vi "DDS220_xc_umn_new.vi"() -> ()   [LabVIEW 2015]
uses:
  <vilib>/Analysis/baseanly.llb/Mean (DBL).vi
  <vilib>/Instr/_visa.llb/VISA Configure Serial Port (Instr).vi
  Pixis_FSRS_new/Labview VIs/Stanford Research 830/Public/Data/Read (1 Parameter).vi
  <vilib>/Utility/file.llb/Write To Spreadsheet File (DBL).vi
  <vilib>/Analysis/NI_AALBase.lvlib
  Pixis_FSRS_new/Labview VIs/Stanford Research 830/Stanford Research 830.lvlib
panel:
  in  "Vy input":dbl
  in  "Vx input":dbl
  in  "Move 2D Mirror":bool
  in  "MG17Motor":refnum<k7>(container)
  in  "Serial":i32=94868093
  out "Thor error in readout":errorcluster
  in  "Thor error in (no error)":errorcluster
  out "Boolean":bool
  out "Waveform Graph":dbl[](graph)=[-3.576299999999999e-07, 9.735509166666665e-07, -8.543369166666667e-07, -1.3311782499999997e-06, 2.582899166666667e-07, -1.5497290833333338e-06, 3.715376083333334e-06, -9.934158333333333e-07, -6.159184166666667e-07, -7.947341666666668e-07, -5.960483333333331e-07, -6.357897500000001e-07, -8.543380833333334e-07, 3.377623333333333e-07, -4.967065833333332e-07, -7.748691666666666e-07, -1.1126248333333334e-06, 1.3113100833333334e-06, -1.6888085833333337e-06, -8.145998333333333e-07, -1.7086741666666665e-06, 1.45038675e-06, -1.033152583333333e-06, -7.152597500000001e-07, -8.543379999999999e-07, 7.549975833333334e-07, 2.0663075833333334e-06, -1.7682825000000001e-06, -3.1789166666666676e-07, 9.934167499999999e-07, 1.8080217499999998e-06, -1.4305205000000001e-06, -7.3512925e-07, 2.3444625e-06, -5.761805833333333e-07, 2.0861760000000002e-06, 5.761800000000001e-07, 4.0332687499999995e-06, 1.0530233333333335e-06, 1.1523649166666668e-06, 1.1921008333333334e-06, -1.7881241666666663e-07, 2.2252532499999997e-06, 4.768409166666669e-07, 2.185515833333333e-06, 2.3245900833333336e-06, 4.5697000000000005e-07, 1.2119715833333334e-06, -8.146023333333334e-07, 1.7484133333333331e-06, 3.6359025833333332e-06, 2.980246e-06, 1.7285456666666667e-06, 2.8212999999999996e-06, 5.086294e-06, 4.808134083333333e-06, 3.814720916666667e-06, 4.768400833333334e-06, 4.669061000000001e-06, 5.6624715e-06, 7.212209166666667e-06, 1.1364680000000002e-05, 7.967199166666664e-06, 9.199042499999999e-06, 1.0311664166666666e-05, 1.4484019166666666e-05, 1.6093358333333332e-05, 2.0603458333333332e-05, 2.094121666666667e-05, 2.4616841666666666e-05, 2.870973333333333e-05, 2.8828933333333334e-05, 3.323970833333333e-05, 3.6935225e-05, 4.146518333333334e-05, 4.456464166666667e-05, 5.8452574999999995e-05, 6.701593333333332e-05, 8.302974166666666e-05, 9.667923333333334e-05, 0.00010430865, 0.00011529566666666664, 0.00013200541666666667, 0.00014907225000000002, 0.00016401308333333333, 0.00017162258333333334, 0.00018302691666666662, 0.00017992758333333332, 0.00016901983333333332, 0.00015932408333333334, 0.00014724416666666665, 0.00013774725, 0.00012362083333333331, 0.00011342816666666667, 0.00010422908333333334, 8.1599225e-05, 6.351909166666666e-05, 5.539285833333333e-05, 4.4524900000000005e-05, 3.888233333333333e-05, 3.757101666666667e-05, 3.92797e-05, 3.643850833333333e-05, 3.0795925e-05, 2.5669866666666666e-05, 2.0166358333333336e-05, 1.8159649999999995e-05, 1.3272034166666667e-05, 1.3788616666666667e-05, 1.38879575e-05, 1.4742300000000001e-05, 1.0808380833333335e-05, 8.2850935e-06, 9.556669166666668e-06, 7.410888333333332e-06, 6.258529166666666e-06, 4.271688416666667e-06, 5.9406249999999996e-06, 5.920766666666666e-06, 3.2186668333333334e-06, 3.9537975e-06, 6.794973250000001e-06, 6.238653333333333e-06, 5.1657625000000005e-06, 2.3643309166666665e-06, 1.966964e-06, 3.7948526666666665e-06, 5.304841833333333e-06, 4.311425083333332e-06, 3.616038416666667e-06, 2.40406775e-06, 1.6888091666666666e-06, 4.212084333333333e-06, 3.178937666666667e-06, 3.0398556666666672e-06, 1.3709143333333332e-06, 7.152594999999999e-07, 2.284862666666667e-06, 8.146010833333332e-07, 1.9272292499999995e-06, 2.1259103333333337e-06, 3.159062666666667e-06, -5.36446e-07, 1.0132839999999999e-06, 1.0728908333333333e-06, -5.165766666666667e-07, 1.5497284999999996e-06, 1.1722341666666662e-06, 3.794851750000001e-06, 3.973675000000048e-08, 1.0728899999999999e-06, 1.0530215833333335e-06, 1.2715725833333337e-06, 2.4636706666666665e-06, 2.1060426666666664e-06, -2.384209166666666e-07, 1.9868385833333334e-06, 3.3577483333333332e-06, 3.9736666666666353e-08, -6.755207499999998e-07, 2.0066975833333333e-06, 3.9736645e-06, 8.344708333333334e-07, 3.0994578333333333e-06, 1.5298624166666668e-06, 2.4835408333333335e-06, 2.145781e-06, 2.88090675e-06, 2.8809068333333336e-06, 1.1920974999999993e-07, 3.5564320833333337e-06, 2.7815666666666668e-06, 2.1259160000000003e-06, 8.940750000000001e-07, -2.76169575e-06, 3.6756387499999998e-06, 5.761815833333333e-07, -8.146014166666668e-07, 8.940749999999999e-07, -1.788150833333334e-07, -9.338119166666668e-07, 1.0927573333333334e-06, 1.27157425e-06, -1.1722292500000002e-06, 1.2318368333333332e-06, -4.172325e-07, 2.2848560000000004e-06, 1.3709118333333336e-06, 2.7616977500000003e-06, 3.337880083333333e-06, -9.934159166666668e-07, -1.5894266666666665e-07, 3.7749766666666664e-07, -7.152651666666667e-07, 9.139435833333334e-07, -1.986808333333333e-08, -4.3710175000000006e-07, 1.5298618333333338e-06, -1.291440833333333e-06, 1.2715725000000002e-06]
  in  "Shutter Position":bool=TRUE
  out "Status":string="Shutter Open"
  out "Numeric 2":i32=1
  in  "error out 3":errorcluster
  out "error out 2":errorcluster
  out "Current position":dbl=18.1998
  in  "move":bool
  in  "flow control 2":u16(ring) items=["None"=0, "XON/XOFF"=1, "RTS/CTS"=2, "DTR/DSR"=4]
  in  "stop bits 2":u16(ring)=10 items=["1.0"=10, "1.5"=15, "2.0"=20]
  in  "parity 2":u16(ring) items=["None", "Odd", "Even", "Mark", "Space"]
  in  "data bits 2":u16=8 min=5 max=8 step=1
  in  "VISA resource name 3":refnum<visa-resource-name>="GPIB0::8::INSTR"
  in  "baud rate 2":u32=9600
  in  "Start Position":dbl=17.8
  out "read buffer":string="-2.86104e-006\r"
  out "Numeric":dbl=14.0
  out "Array 2":dbl[](array[numeric])=[17.8019, 17.8038, 17.8058, 17.8078, 17.8098, 17.8118, 17.8138, 17.8157, 17.8177, 17.8199, 17.8219, 17.8237, 17.8258, 17.8278, 17.8298, 17.8318, 17.8337, 17.8358, 17.8378, 17.8398, 17.8418, 17.8438, 17.8458, 17.8478, 17.8497, 17.8518, 17.8538, 17.8558, 17.8578, 17.8598, 17.8618, 17.8638, 17.8658, 17.8678, 17.8698, 17.8718, 17.8737, 17.8759, 17.8778, 17.8799, 17.8818, 17.8838, 17.8858, 17.8878, 17.8898, 17.8918, 17.8938, 17.8958, 17.8978, 17.8996, 17.9018, 17.9038, 17.9058, 17.9077, 17.9098, 17.9118, 17.9138, 17.9159, 17.9177, 17.9197, 17.9218, 17.9238, 17.9258, 17.9278, 17.9298, 17.9318, 17.9338, 17.9357, 17.9378, 17.9397, 17.9419, 17.9438, 17.9458, 17.9478, 17.9499, 17.9518, 17.9538, 17.9559, 17.9579, 17.9596, 17.9618, 17.9637, 17.9658, 17.9678, 17.9698, 17.9718, 17.9738, 17.9759, 17.9777, 17.9801, 17.9818, 17.9838, 17.9858, 17.9878, 17.9898, 17.9918, 17.9938, 17.9957, 17.9978, 18.0, 18.0018, 18.0038, 18.0057, 18.0078, 18.0098, 18.0118, 18.0138, 18.0157, 18.0178, 18.0199, 18.0218, 18.0238, 18.0258, 18.0278, 18.0298, 18.0318, 18.0338, 18.0358, 18.0378, 18.0401, 18.0418, 18.0438, 18.0458, 18.0478, 18.0498, 18.0518, 18.0538, 18.0557, 18.0578, 18.06, 18.0618, 18.0638, 18.0658, 18.0677, 18.0698, 18.0718, 18.0738, 18.0758, 18.0778, 18.0796, 18.0818, 18.0838, 18.0857, 18.0878, 18.0898, 18.0918, 18.0937, 18.0958, 18.0978, 18.0998, 18.1018, 18.1038, 18.1058, 18.1078, 18.1098, 18.1118, 18.1138, 18.1159, 18.1178, 18.1198, 18.1218, 18.1237, 18.1257, 18.1277, 18.1297, 18.1318, 18.1338, 18.1356, 18.1378, 18.1398, 18.1418, 18.1437, 18.1457, 18.1478, 18.1498, 18.1518, 18.1538, 18.1558, 18.1577, 18.1598, 18.1618, 18.1637, 18.1658, 18.1678, 18.1698, 18.1718, 18.1738, 18.1758, 18.1778, 18.1798, 18.1818, 18.1838, 18.1858, 18.1878, 18.1898, 18.1917, 18.1937, 18.1958, 18.1977, 18.1998]
  out "Array":dbl[](array[numeric])=[-3.576299999999999e-07, 9.735509166666665e-07, -8.543369166666667e-07, -1.3311782499999997e-06, 2.582899166666667e-07, -1.5497290833333338e-06, 3.715376083333334e-06, -9.934158333333333e-07, -6.159184166666667e-07, -7.947341666666668e-07, -5.960483333333331e-07, -6.357897500000001e-07, -8.543380833333334e-07, 3.377623333333333e-07, -4.967065833333332e-07, -7.748691666666666e-07, -1.1126248333333334e-06, 1.3113100833333334e-06, -1.6888085833333337e-06, -8.145998333333333e-07, -1.7086741666666665e-06, 1.45038675e-06, -1.033152583333333e-06, -7.152597500000001e-07, -8.543379999999999e-07, 7.549975833333334e-07, 2.0663075833333334e-06, -1.7682825000000001e-06, -3.1789166666666676e-07, 9.934167499999999e-07, 1.8080217499999998e-06, -1.4305205000000001e-06, -7.3512925e-07, 2.3444625e-06, -5.761805833333333e-07, 2.0861760000000002e-06, 5.761800000000001e-07, 4.0332687499999995e-06, 1.0530233333333335e-06, 1.1523649166666668e-06, 1.1921008333333334e-06, -1.7881241666666663e-07, 2.2252532499999997e-06, 4.768409166666669e-07, 2.185515833333333e-06, 2.3245900833333336e-06, 4.5697000000000005e-07, 1.2119715833333334e-06, -8.146023333333334e-07, 1.7484133333333331e-06, 3.6359025833333332e-06, 2.980246e-06, 1.7285456666666667e-06, 2.8212999999999996e-06, 5.086294e-06, 4.808134083333333e-06, 3.814720916666667e-06, 4.768400833333334e-06, 4.669061000000001e-06, 5.6624715e-06, 7.212209166666667e-06, 1.1364680000000002e-05, 7.967199166666664e-06, 9.199042499999999e-06, 1.0311664166666666e-05, 1.4484019166666666e-05, 1.6093358333333332e-05, 2.0603458333333332e-05, 2.094121666666667e-05, 2.4616841666666666e-05, 2.870973333333333e-05, 2.8828933333333334e-05, 3.323970833333333e-05, 3.6935225e-05, 4.146518333333334e-05, 4.456464166666667e-05, 5.8452574999999995e-05, 6.701593333333332e-05, 8.302974166666666e-05, 9.667923333333334e-05, 0.00010430865, 0.00011529566666666664, 0.00013200541666666667, 0.00014907225000000002, 0.00016401308333333333, 0.00017162258333333334, 0.00018302691666666662, 0.00017992758333333332, 0.00016901983333333332, 0.00015932408333333334, 0.00014724416666666665, 0.00013774725, 0.00012362083333333331, 0.00011342816666666667, 0.00010422908333333334, 8.1599225e-05, 6.351909166666666e-05, 5.539285833333333e-05, 4.4524900000000005e-05, 3.888233333333333e-05, 3.757101666666667e-05, 3.92797e-05, 3.643850833333333e-05, 3.0795925e-05, 2.5669866666666666e-05, 2.0166358333333336e-05, 1.8159649999999995e-05, 1.3272034166666667e-05, 1.3788616666666667e-05, 1.38879575e-05, 1.4742300000000001e-05, 1.0808380833333335e-05, 8.2850935e-06, 9.556669166666668e-06, 7.410888333333332e-06, 6.258529166666666e-06, 4.271688416666667e-06, 5.9406249999999996e-06, 5.920766666666666e-06, 3.2186668333333334e-06, 3.9537975e-06, 6.794973250000001e-06, 6.238653333333333e-06, 5.1657625000000005e-06, 2.3643309166666665e-06, 1.966964e-06, 3.7948526666666665e-06, 5.304841833333333e-06, 4.311425083333332e-06, 3.616038416666667e-06, 2.40406775e-06, 1.6888091666666666e-06, 4.212084333333333e-06, 3.178937666666667e-06, 3.0398556666666672e-06, 1.3709143333333332e-06, 7.152594999999999e-07, 2.284862666666667e-06, 8.146010833333332e-07, 1.9272292499999995e-06, 2.1259103333333337e-06, 3.159062666666667e-06, -5.36446e-07, 1.0132839999999999e-06, 1.0728908333333333e-06, -5.165766666666667e-07, 1.5497284999999996e-06, 1.1722341666666662e-06, 3.794851750000001e-06, 3.973675000000048e-08, 1.0728899999999999e-06, 1.0530215833333335e-06, 1.2715725833333337e-06, 2.4636706666666665e-06, 2.1060426666666664e-06, -2.384209166666666e-07, 1.9868385833333334e-06, 3.3577483333333332e-06, 3.9736666666666353e-08, -6.755207499999998e-07, 2.0066975833333333e-06, 3.9736645e-06, 8.344708333333334e-07, 3.0994578333333333e-06, 1.5298624166666668e-06, 2.4835408333333335e-06, 2.145781e-06, 2.88090675e-06, 2.8809068333333336e-06, 1.1920974999999993e-07, 3.5564320833333337e-06, 2.7815666666666668e-06, 2.1259160000000003e-06, 8.940750000000001e-07, -2.76169575e-06, 3.6756387499999998e-06, 5.761815833333333e-07, -8.146014166666668e-07, 8.940749999999999e-07, -1.788150833333334e-07, -9.338119166666668e-07, 1.0927573333333334e-06, 1.27157425e-06, -1.1722292500000002e-06, 1.2318368333333332e-06, -4.172325e-07, 2.2848560000000004e-06, 1.3709118333333336e-06, 2.7616977500000003e-06, 3.337880083333333e-06, -9.934159166666668e-07, -1.5894266666666665e-07, 3.7749766666666664e-07, -7.152651666666667e-07, 9.139435833333334e-07, -1.986808333333333e-08, -4.3710175000000006e-07, 1.5298618333333338e-06, -1.291440833333333e-06, 1.2715725000000002e-06]
  in  "Averages":u16=12
  out "error out":errorcluster
  in  "error in":errorcluster
  in  "save":bool
  out "Current Mean":dbl=1.2715725000000002e-06
  in  "quit Button":bool
  in  "Start Button":bool
  in  "Increment (in mm)":dbl=0.002
  in  "Range (in mm)":dbl=0.4
  # "Before you start any scan, scroll to your\nleft and click on the home button, so \nthat our ThorLabs stage will move to its\nhome position (middle).\n\nIt's controlled via Active X. so you can \ninteract with the panel."
  # "Used to control 2D mirror positions.\nIgnore if not relevant. Doesn't interfere\nwith Kerr measurement."
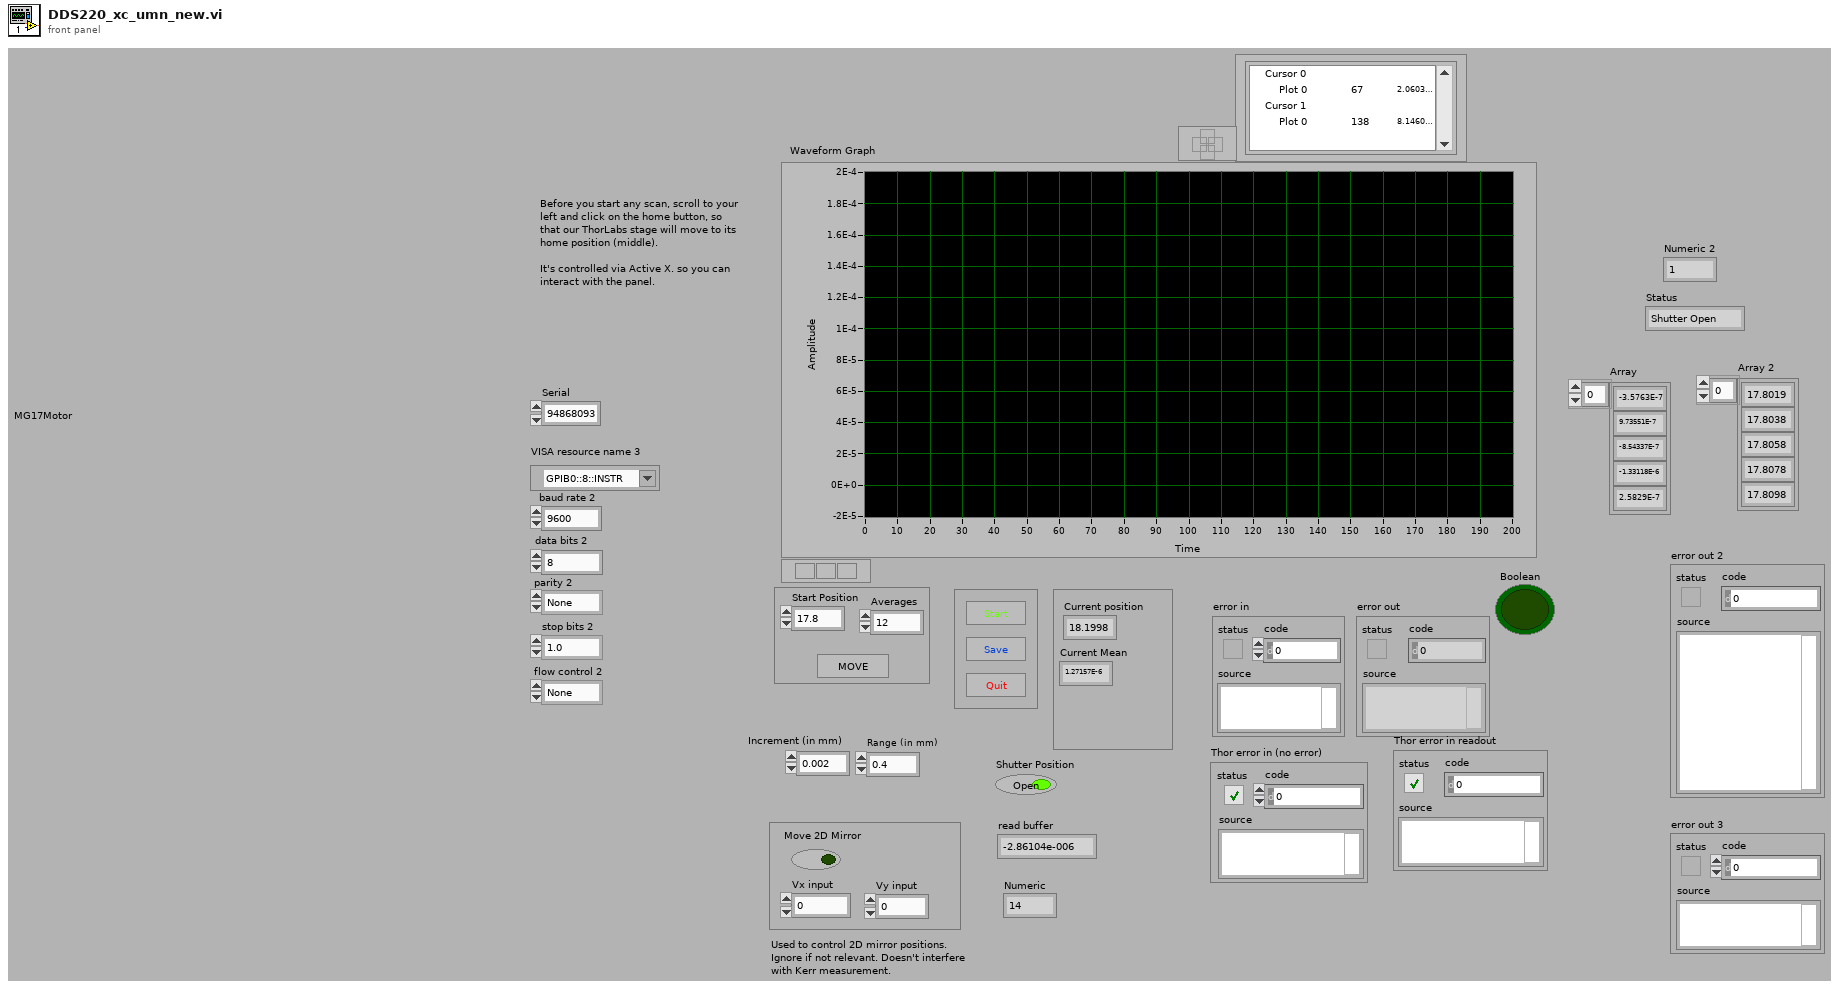
[diagram p1: front panel]
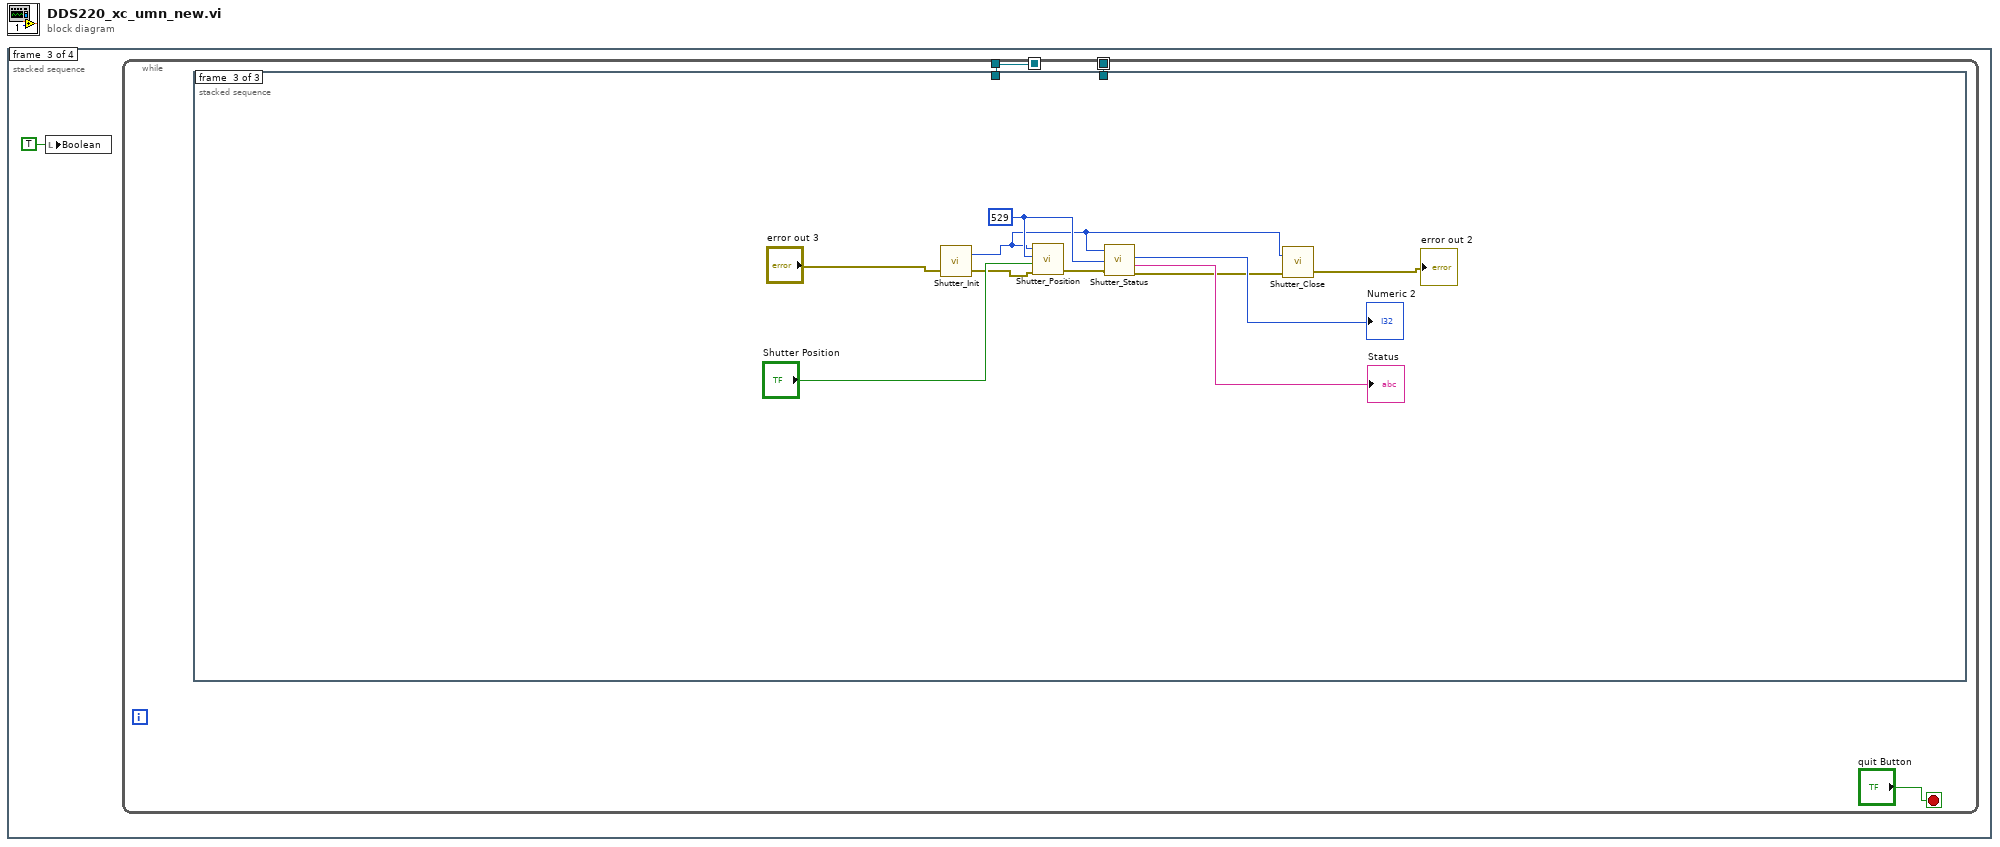
[diagram p0: block diagram]
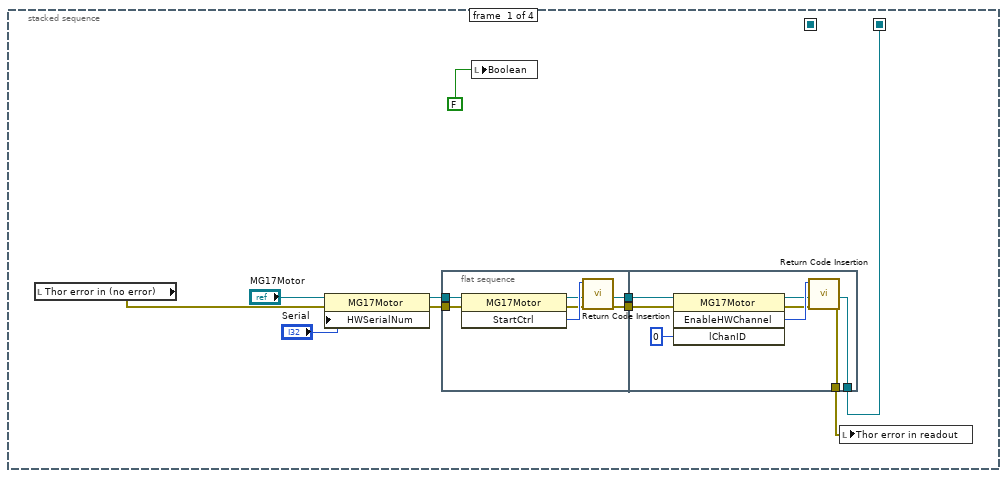
[diagram p2: hidden frame]
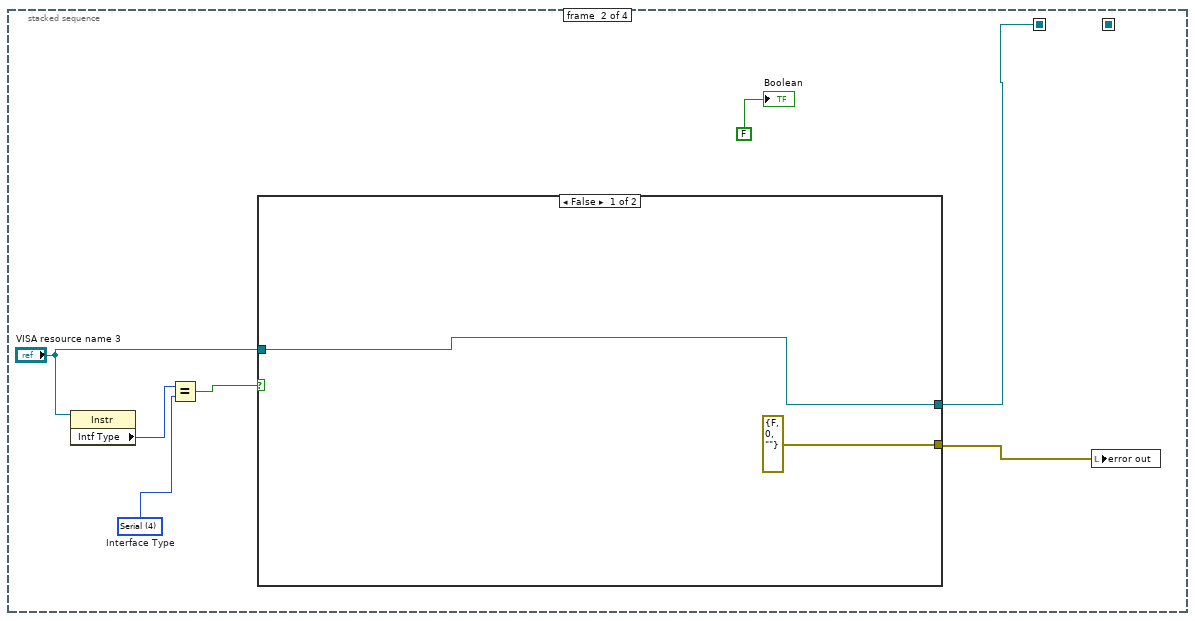
[diagram p3: hidden frame]
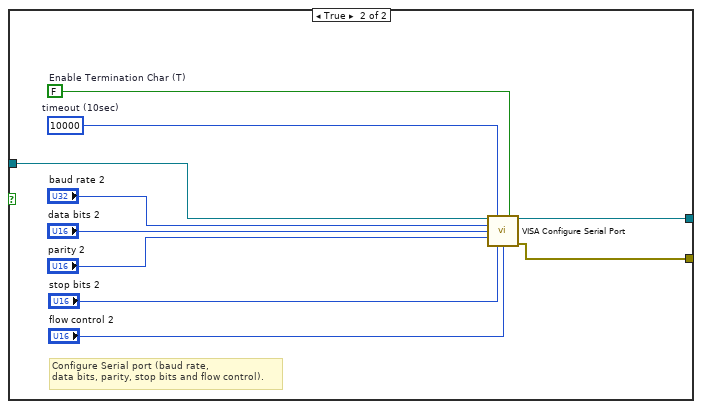
[diagram p4: hidden frame]
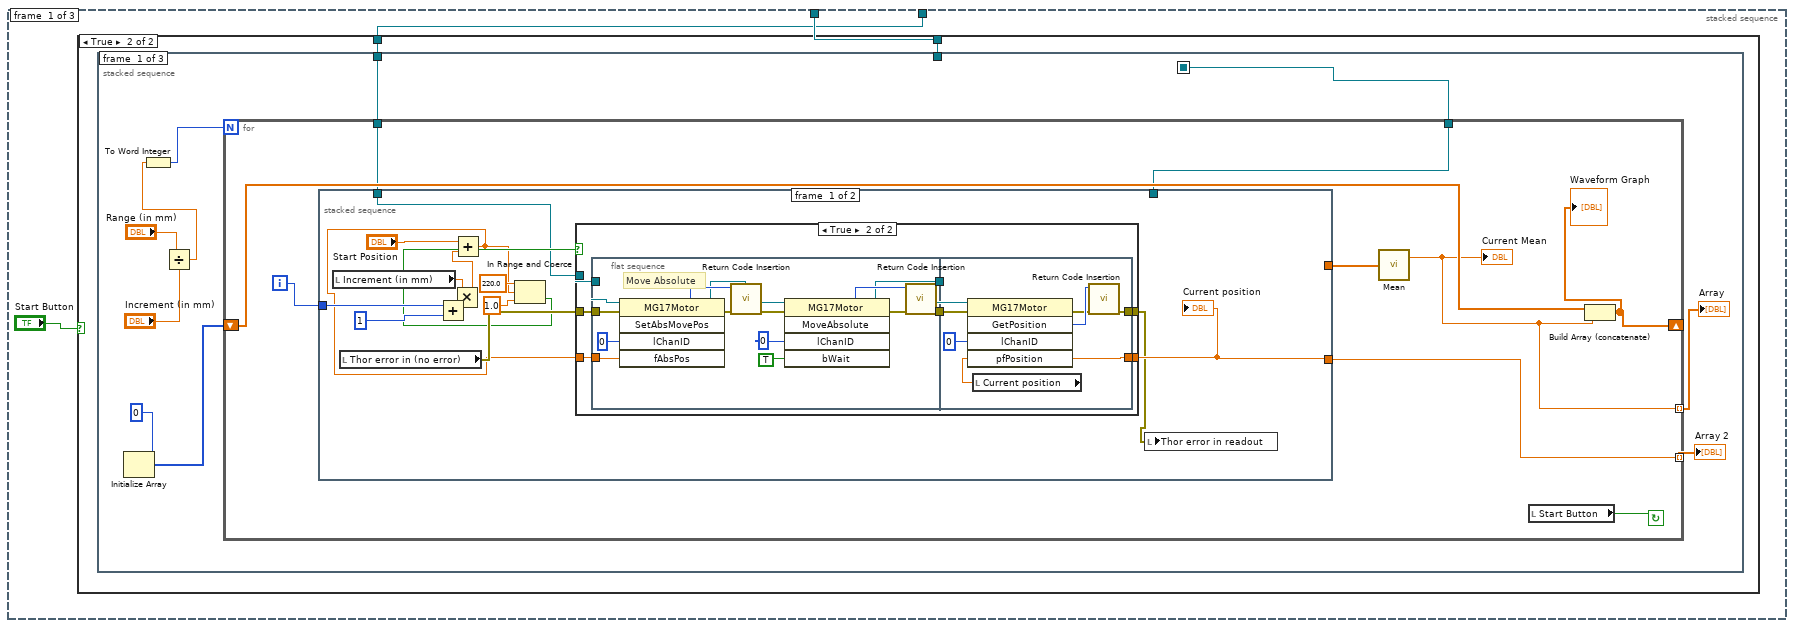
[diagram p5: hidden frame]
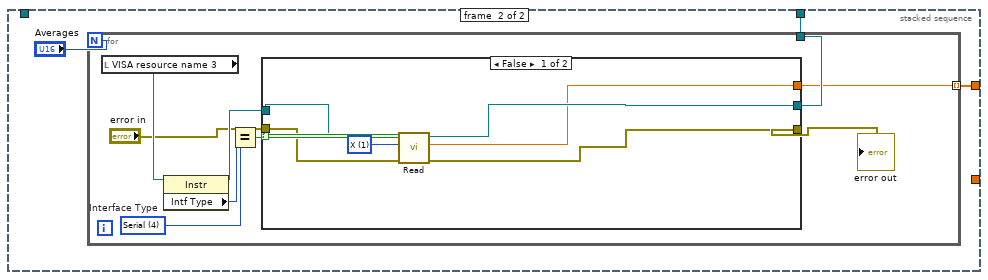
[diagram p8: hidden frame]
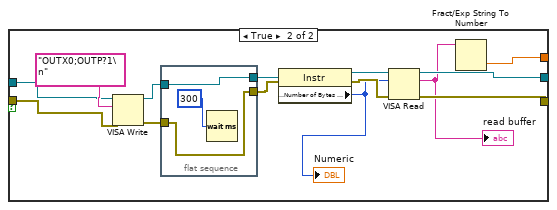
[diagram p9: hidden frame]
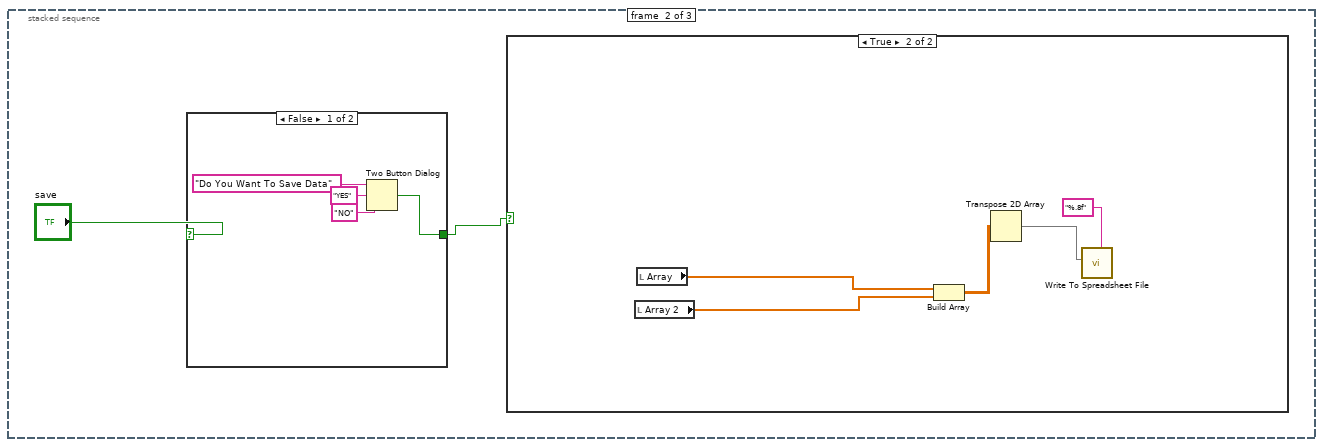
[diagram p10: hidden frame]
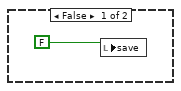
[diagram p12: hidden frame]
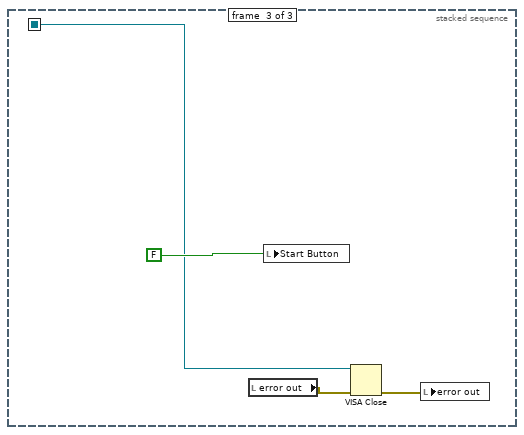
[diagram p13: hidden frame]
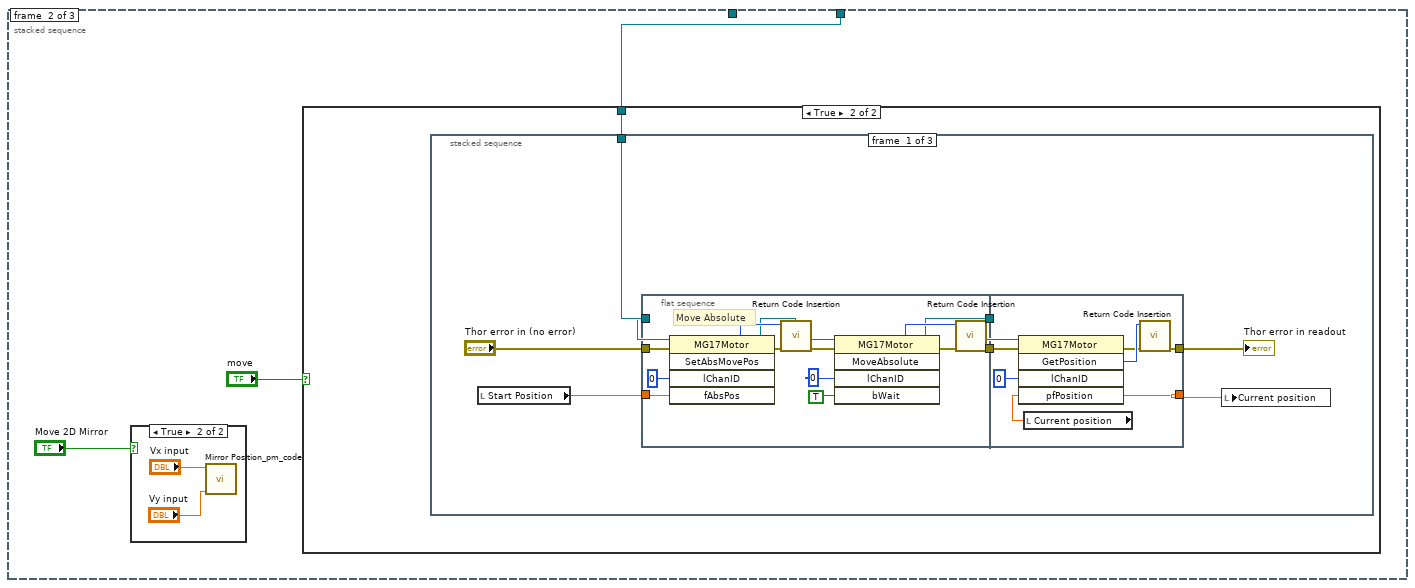
[diagram p14: hidden frame]
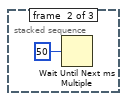
[diagram p17: hidden frame]
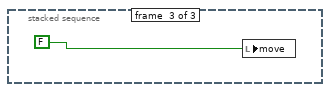
[diagram p18: hidden frame]
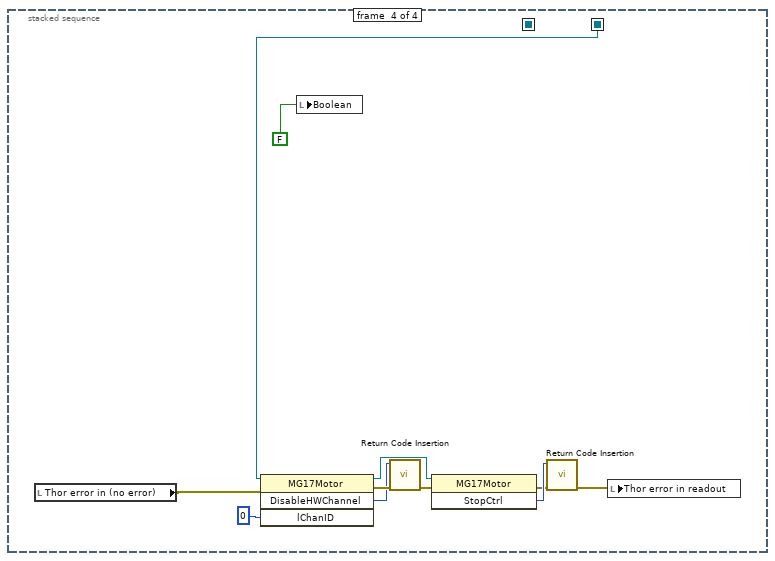
[diagram p19: hidden frame]
diagram:
  n1 = stacked-sequence {
    seq-local: [_ w30 _ _] -> [_ _ w45 _]
    seq-local: [w3 _ _ _] -> [_ _ w43 w217]
    frame #0 {
      n2 = local read "Thor error in (no error)"() -> (w2:errorcluster)
      n3 = property class="MG17Motor"(reference="MG17Motor", error in=w2, "HWSerialNum"="Serial") -> (reference out=w5:refnum<k7>, error out=w4:errorcluster)
      n4 = flat-sequence {
        tunnel: w5 -> [w16]
        tunnel: w4 -> [w15]
        tunnel: [w11] -> w9
        tunnel: [w12] -> w8
        tunnel: [w17] -> w1
        tunnel: w9 -> [w18]
        tunnel: w8 -> [w20]
        tunnel: [w19] -> w3
        frame #0 {
          n5 = invoke class="MG17Motor" method="StartCtrl"(reference=w16, error in=w15) -> (reference out=w12:refnum<k7>, error out=w13:errorcluster, "StartCtrl"=w14:i32)  [unwired: 1 in]
          n6 = call "Return Code Insertion.vi"("error in (no error)"=w13, "Return Code"=w14) -> ("error out"=w11:errorcluster)  [unwired: 9 in]
        }
        frame #1 {
          n7 = invoke class="MG17Motor" method="EnableHWChannel"(reference=w20, error in=w18, "lChanID"=0) -> (reference out=w19:refnum<k7>, error out=w21:errorcluster, "EnableHWChannel"=w22:i32)  [unwired: 1 in, 1 out]
          n8 = call "Return Code Insertion.vi"("error in (no error)"=w21, "Return Code"=w22) -> ("error out"=w17:errorcluster)  [unwired: 9 in]
        }
      }
      n9 = local write "Boolean"(FALSE ("Boolean")) -> ()
      n10 = local write "Thor error in readout"(w1) -> ()
    }
    frame #1 {
      w27 = u16 4 items=["GPIB"=1, "VXI"=2, "GPIB-VXI"=3, "Serial"=4, "PXI"=5, "TCPIP"=6, "USB"=7]  # Interface Type
      n11 = property class="Instr"(reference="VISA resource name 3") -> ("Intf Type"=w28:u16)  [unwired: 1 in, 2 out]
      n12 = Equal?(x=w28, y=w27) -> (x = y?=w26:bool)
      n13 = case shown="False" w26 {
        tunnel: [w32 w42] -> w30
        tunnel: [errorcluster {"status"=FALSE, "code"=0, "source"=""} ("error out") w41] -> w24
        tunnel: "VISA resource name 3" -> [w32 w40]
        frame False {
        }
        frame True {
          w36 = FALSE  # Enable Termination Char (T)
          w37 = u32 10000  # timeout (10sec)
          # "Configure Serial port (baud rate,\ndata bits, parity, stop bits and flow control)."
          n14 = call-poly "VISA Configure Serial Port"("VISA resource name"=w40, "timeout (10sec)"=w37, "Enable Termination\nChar (T)"=w36, "baud rate (9600)"="baud rate 2", "data bits (8)"="data bits 2", "parity (0:none)"="parity 2", "stop bits (10: 1 bit)"="stop bits 2", "flow control (0:none)"="flow control 2") -> ("VISA resource name out"=w42:refnum<visa-resource-name>, "error out"=w41:errorcluster)  [unwired: 6 in]
        }
      }
      n15 = local write "error out"(w24) -> ()
      "Boolean" <- FALSE ("Boolean")
    }
    frame #2 {
      n16 = local write "Boolean"(TRUE ("Boolean")) -> ()
      n17 = while {
        tunnel: w45 -> [w47]
        tunnel: w43 -> [w46]
        stop <- "quit Button" stop-if-true
        n18 = stacked-sequence {
          tunnel: w47 -> [w50 _ _]
          tunnel: w46 -> [w49 w171 _]
          frame #0 {
            n19 = case shown="True" "Start Button" {
              tunnel: w50 -> [_ w53]
              tunnel: w49 -> [_ w52]
              frame False {
              }
              frame True {
                n20 = stacked-sequence {
                  seq-local: [w55 _ _] -> [_ _ w166]
                  tunnel: w53 -> [_ _ _]
                  tunnel: w52 -> [w54 _ _]
                  frame #0 {
                    n21 = Initialize Array(0) -> (w58:i32[])  [unwired: 1 in]
                    n22 = Divide(x="Range (in mm)", y="Increment (in mm)") -> (x/y=w61:dbl)
                    n23 = To Word Integer(number=w61) -> (16bit integer=w60:i16)
                    n24 = for {
                      N: w60 -> [_]
                      shift-right: [w67] -> _
                      shift-left: w58 -> [w71]
                      tunnel: [w70] -> w57 mode=indexing
                      tunnel: [w69] -> w56 mode=indexing
                      tunnel: [w68] -> w55
                      tunnel: w54 -> [w64]
                      i -> [w72]
                      stop <- w65 continue-if-true
                      n25 = stacked-sequence {
                        tunnel: w72 -> [w81 _]
                        tunnel: [_ w119] -> w66
                        tunnel: [_ w118] -> w68
                        tunnel: [w75 _] -> w69
                        tunnel: w64 -> [w76 _]
                        frame #0 {
                          n26 = local read "Increment (in mm)"() -> (w83:dbl)
                          n27 = local read "Thor error in (no error)"() -> (w78:errorcluster)
                          n28 = Add(x=w81, y=1) -> (x+y=w84:i32)
                          n29 = Multiply(x=w83, y=w84) -> (x*y=w85:dbl)
                          n30 = Add(x="Start Position", y=w85) -> (x+y=w74:dbl)
                          n31 = In Range and Coerce(upper limit=220.0, x=w74, lower limit=1.0) -> (In Range?=w77:bool)  [unwired: 1 out]
                          n32 = case shown="True" w77 {
                            tunnel: [w88 w93] -> w73
                            tunnel: w76 -> [_ w92]
                            tunnel: w78 -> [w88 w91]
                            tunnel: [w87 w90] -> w75
                            tunnel: w74 -> [w87 w89]
                            frame False {
                            }
                            frame True {
                              n33 = flat-sequence {
                                tunnel: w91 -> [w100]
                                tunnel: w92 -> [w99]
                                tunnel: [w98] -> w95
                                tunnel: [w97] -> w94
                                tunnel: w89 -> [w96]
                                tunnel: w95 -> [w113]
                                tunnel: w94 -> [w112]
                                tunnel: [w111] -> w93
                                tunnel: [w110] -> w90
                                frame #0 {
                                # "Move Absolute"
                                n34 = invoke class="MG17Motor" method="SetAbsMovePos"(reference=w99, error in=w100, "lChanID"=0, "fAbsPos"=w96) -> (reference out=w105:refnum<k7>, error out=w104:errorcluster, "SetAbsMovePos"=w106:i32)  [unwired: 1 in, 2 out]
                                n35 = call "Return Code Insertion.vi"("error in (no error)"=w104, "Return Code"=w106) -> ("error out"=w103:errorcluster)  [unwired: 9 in]
                                n36 = invoke class="MG17Motor" method="MoveAbsolute"(reference=w105, error in=w103, "lChanID"=0, "bWait"=TRUE) -> (reference out=w98:refnum<k7>, error out=w101:errorcluster, "MoveAbsolute"=w102:i32)  [unwired: 1 in, 2 out]
                                n37 = call "Return Code Insertion.vi"("error in (no error)"=w101, "Return Code"=w102) -> ("error out"=w97:errorcluster)  [unwired: 9 in]
                                }
                                frame #1 {
                                n38 = local read "Current position"() -> (w116:dbl)
                                n39 = invoke class="MG17Motor" method="GetPosition"(reference=w113, error in=w112, "lChanID"=0, "pfPosition"=w116) -> (error out=w114:errorcluster, "GetPosition"=w115:i32, "pfPosition"=w110:sgl)  [unwired: 1 in, 2 out]
                                n40 = call "Return Code Insertion.vi"("error in (no error)"=w114, "Return Code"=w115) -> ("error out"=w111:errorcluster)  [unwired: 9 in]
                                }
                              }
                            }
                          }
                          "Current position" <- w75
                          n41 = local write "Thor error in readout"(w73) -> ()
                        }
                        frame #1 {
                          n42 = for {
                            N: "Averages" -> [_]
                            tunnel: [w121] -> w119 mode=indexing
                            tunnel: [w123] -> w118
                            w126 = u16 4 items=["GPIB"=1, "VXI"=2, "GPIB-VXI"=3, "Serial"=4, "PXI"=5, "TCPIP"=6, "USB"=7]  # Interface Type
                            n43 = local read "VISA resource name 3"() -> (w129:refnum<visa-resource-name>)
                            n44 = property class="Instr"(reference=w129) -> (reference out=w125:refnum<visa-resource-name>, "Intf Type"=w127:u16)  [unwired: 1 in, 1 out]
                            n45 = Equal?(x=w127, y=w126) -> (x = y?=w128:bool)
                            n46 = case shown="False" w128 {
                              tunnel: w125 -> [w134 w148]
                              tunnel: "error in" -> [w135 w147]
                              tunnel: [w133 w141] -> w123
                              tunnel: [w132 w139] -> w122
                              tunnel: [w131 w138] -> w121
                              frame False {
                                w130 = u16 1 items=["X"=1, "Y"=2, "R"=3, "Theta"=4, "Channel 1"=5, "Channel 2"=6, "Aux In 1"=7, "Aux In 2"=8, "Aux In 3"=9, "Aux In 4"=10] ("Parameter (1: X)")
                                n47 = call-poly "Read.vi"("error in (no error)"=w135, "Parameter (1: X)"=w130, "VISA resource name"=w134) -> ("error out"=w132:errorcluster, "Measurement"=w131:dbl, "VISA resource name out"=w133:refnum<visa-resource-name>)  [unwired: 6 in]
                              }
                              frame True {
                                n48 = VISA Write(VISA resource name=w148, write buffer="OUTX0;OUTP?1\n" ("string to write"), error in (no error)=w147) -> (VISA resource name out=w146:refnum<visa-resource-name>, error out=w144:errorcluster)  [unwired: 1 out]
                                n49 = flat-sequence {
                                tunnel: [w151] -> w145
                                tunnel: w146 -> [w151]
                                tunnel: [w150] -> w143
                                tunnel: w144 -> [w150]
                                frame #0 {
                                n50 = Wait (ms)(milliseconds to wait=300) -> ()  [unwired: 1 out]
                                }
                                }
                                n51 = property class="Instr"(reference=w145, error in=w143) -> (reference out=w142:refnum<visa-resource-name>, error out=w140:errorcluster, "Serial Settings:Number of Bytes at Serial Port"=w136:u32)
                                "Numeric" <- w136
                                n52 = VISA Read(VISA resource name=w142, byte count=w136, error in (no error)=w140) -> (VISA resource name out=w141:refnum<visa-resource-name>, read buffer=w137:string, error out=w139:errorcluster)  [unwired: 1 out]
                                "read buffer" <- w137
                                n53 = Fract/Exp String To Number(string=w137) -> (number=w138:dbl)  [unwired: 3 in, 1 out]
                              }
                            }
                            "error out" <- w122
                          }
                        }
                      }
                      n54 = call-poly <vilib>:"Mean.vi"("X"=w66) -> ("mean"=w70:dbl)  [unwired: 1 out]
                      "Current Mean" <- w70
                      n55 = local read "Start Button"() -> (w65:bool)
                      n56 = Build Array (concatenate)(w71, w70) -> (w67:dbl[])
                      "Waveform Graph" <- w67
                    }
                    "Array" <- w57
                    "Array 2" <- w56
                  }
                  frame #1 {
                    n57 = case shown="False" "save" {
                      selector: "save" -> [_ w159]
                      tunnel: [w155 w159] -> w153
                      frame False {
                        n58 = Two Button Dialog(message="Do You Want To Save Data", 1:"NO" ("F button name (\"Cancel\")"), 2:"YES" ("T button name (\"OK\")")) -> (T button?=w155:bool)
                      }
                      frame True {
                      }
                    }
                    n59 = case shown="True" w153 {
                      frame False {
                        n60 = local write "save"(FALSE) -> ()
                      }
                      frame True {
                        n61 = local read "Array 2"() -> (w161:dbl[])
                        n62 = local read "Array"() -> (w162:dbl[])
                        n63 = Build Array(w162, w161) -> (w164:dbl[][])
                        n64 = Transpose 2D Array(2D array=w164) -> (transposed array=w163:dbl[][])
                        n65 = call-poly <vilib>:"Write To Spreadsheet File.vi"("format (%.5f)"="%.8f", "2D data"=w163) -> ()  [unwired: 6 in, 1 out]
                      }
                    }
                  }
                  frame #2 {
                    n66 = local read "error out"() -> (w168:errorcluster)
                    n67 = local write "Start Button"(FALSE) -> ()
                    n68 = VISA Close(VISA resource name=w166, error in (no error)=w168) -> (error out=w167:errorcluster)
                    n69 = local write "error out"(w167) -> ()
                  }
                }
              }
            }
          }
          frame #1 {
            n70 = case shown="True" "Move 2D Mirror" {
              frame False {
              }
              frame True {
                n71 = call "Mirror Position_pm_code.vi"("Analog O/p 1"="Vy input", "Analog O/p 0"="Vx input") -> ()  [unwired: 8 in]
              }
            }
            n72 = case shown="True" "move" {
              tunnel: w171 -> [_ w175]
              frame False {
              }
              frame True {
                n73 = stacked-sequence {
                  tunnel: w175 -> [w179 _ _]
                  frame #0 {
                    n74 = local read "Start Position"() -> (w178:dbl)
                    n75 = flat-sequence {
                      tunnel: "Thor error in (no error)" -> [w187]
                      tunnel: w179 -> [w186]
                      tunnel: [w185] -> w177
                      tunnel: [w184] -> w176
                      tunnel: w178 -> [w183]
                      tunnel: w177 -> [w200]
                      tunnel: w176 -> [w199]
                      tunnel: [w198] -> w181
                      tunnel: [w197] -> w182
                      frame #0 {
                        # "Move Absolute"
                        n76 = invoke class="MG17Motor" method="SetAbsMovePos"(reference=w186, error in=w187, "lChanID"=0, "fAbsPos"=w183) -> (reference out=w192:refnum<k7>, error out=w191:errorcluster, "SetAbsMovePos"=w193:i32)  [unwired: 1 in, 2 out]
                        n77 = call "Return Code Insertion.vi"("error in (no error)"=w191, "Return Code"=w193) -> ("error out"=w190:errorcluster)  [unwired: 9 in]
                        n78 = invoke class="MG17Motor" method="MoveAbsolute"(reference=w192, error in=w190, "lChanID"=0, "bWait"=TRUE) -> (reference out=w185:refnum<k7>, error out=w188:errorcluster, "MoveAbsolute"=w189:i32)  [unwired: 1 in, 2 out]
                        n79 = call "Return Code Insertion.vi"("error in (no error)"=w188, "Return Code"=w189) -> ("error out"=w184:errorcluster)  [unwired: 9 in]
                      }
                      frame #1 {
                        n80 = local read "Current position"() -> (w203:dbl)
                        n81 = invoke class="MG17Motor" method="GetPosition"(reference=w200, error in=w199, "lChanID"=0, "pfPosition"=w203) -> (error out=w201:errorcluster, "GetPosition"=w202:i32, "pfPosition"=w197:sgl)  [unwired: 1 in, 2 out]
                        n82 = call "Return Code Insertion.vi"("error in (no error)"=w201, "Return Code"=w202) -> ("error out"=w198:errorcluster)  [unwired: 9 in]
                      }
                    }
                    n83 = local write "Current position"(w182) -> ()
                    "Thor error in readout" <- w181
                  }
                  frame #1 {
                    n84 = Wait Until Next ms Multiple(millisecond multiple=u32 50) -> ()  [unwired: 1 out]
                  }
                  frame #2 {
                    n85 = local write "move"(FALSE) -> ()
                  }
                }
              }
            }
          }
          frame #2 {
            w212 = 529
            n86 = call "Shutter_Init.vi"("error in"="error out 3") -> ("error out"=w214:errorcluster, "ObjectPtr"=w208:i32)  [unwired: 1 in]
            n87 = call "Shutter_Position.vi"("error in"=w214, "Shutter Position"="Shutter Position", "ShutterID"=w212, "ObjectPtr"=w208) -> ("error out"=w213:errorcluster)  [unwired: 2 in]
            n88 = call "Shutter_Status.vi"("ObjectPtr"=w208, "ShutterID"=w212, "error in"=w213) -> ("Position"=→"Numeric 2":i32, "Status"=→"Status":string, "error out"=w209:errorcluster)  [unwired: 1 out]
            n89 = call "Shutter_Close.vi"("error in"=w209, "ObjectPtr"=w208) -> ("error out"=→"error out 2":errorcluster)  [unwired: 1 in]
          }
        }
      }
    }
    frame #3 {
      n90 = local read "Thor error in (no error)"() -> (w218:errorcluster)
      n91 = invoke class="MG17Motor" method="DisableHWChannel"(reference=w217, error in=w218, "lChanID"=0) -> (reference out=w221:refnum<k7>, error out=w223:errorcluster, "DisableHWChannel"=w222:i32)  [unwired: 1 in, 1 out]
      n92 = local write "Boolean"(FALSE ("Boolean")) -> ()
      n93 = call "Return Code Insertion.vi"("error in (no error)"=w223, "Return Code"=w222) -> ("error out"=w220:errorcluster)  [unwired: 9 in]
      n94 = invoke class="MG17Motor" method="StopCtrl"(reference=w221, error in=w220) -> (error out=w225:errorcluster, "StopCtrl"=w226:i32)  [unwired: 1 in, 1 out]
      n95 = call "Return Code Insertion.vi"("error in (no error)"=w225, "Return Code"=w226) -> ("error out"=w219:errorcluster)  [unwired: 9 in]
      n96 = local write "Thor error in readout"(w219) -> ()
    }
  }
